vi "imp_test_v10_p1.vi"() -> ()   [LabVIEW 2014]
uses:
  <vilib>/LabVIEW Targets/FPGA/cRIO/shared/nicrio_ModuleControls/nicrio_cRIO-9237_DataRatesRing.ctl
  <vilib>/LabVIEW Targets/FPGA/cRIO/shared/nicrio_ModuleControls/nicrio_cRIO-9237_ExcitationVoltageRing.ctl
  <vilib>/rvi/FXPMathLib/FxpSinAndCos/subVIs/nifxpmath_SinAndCos_SimConfig.ctl
  <vilib>/rvi/Emulation/niFpgaGetClockAttributes.vi
  <vilib>/rvi/Emulation/niFpgaSctlEmulationGetInTimedLoop.vi
  <vilib>/rvi/Emulation/niFpgaEmulationReportErrorSimple.vi
  <vilib>/rvi/Emulation/niFpgaProcessEmulError.vi
  <vilib>/rvi/interface/RandomDataEmulation/nirviRandomDataMultiElementFPGAFIFO.vi
  <instcachedir>/0/nirviRandomDataMultiElementFPGAFIFO_AD0CFC12EF974623A9C2E4184BC062B2.lvgen/nirviRandomDataMultiElementFPGAFIFO_AD0CFC12EF974623A9C2E4184BC062B2_028.vi
  <vilib>/rvi/interface/RandomDataEmulation/niFpgaRandomDataHandleErrors.vi
  <vilib>/rvi/Emulation/niFpgaCriticalErrorInLSC.vi
  <vilib>/rvi/FXPMathLib/FxpSinAndCos/simVIs/DllFxpSinAndCosTemp_sub.vi
  <vilib>/rvi/eio/common/nirviEmuTemplateMethod_errors.vi
  <vilib>/rvi/eio/common/nirviEmuTemplatePropertySet_errors.vi
  <vilib>/rvi/DataTransferAndStorage/Container/XNode/niFpgaContainer.xnode
  <vilib>/rvi/interface/RandomDataEmulation/nirviRandomDataFpgaMultiElementTemplate.vi
  <vilib>/rvi/Analysis/measure/butterworth/XNode/niFpgaButterworthFilter.xnode
  <vilib>/rvi/FXPMathLib/FxpSinAndCos/XNode/nifxpmath_SinAndCos.xnode
  <vilib>/eio/EIONode/EIONode.xnode
  <vilib>/eio/EIOPropertyNode/EIOPropertyNode.xnode
  <vilib>/rvi/eio/common/nirviEmuTemplatePropertyGet_errors.vi
  <vilib>/rvi/eio/common/nirviEmuTemplatePropertyGet_noerrors.vi
  <vilib>/rvi/eio/common/nirviEmuTemplatePropertySet_noerrors.vi
panel:
  in  "F_Threshold_p":fxp<+,12,4>
  out "omega_p (Mavg)":fxp<+/-,36,13>
  out "Dp_d (Mavg)":fxp<+/-,36,13>
  out "omega_p2 (Mavg)":fxp<+/-,36,14>
  out "Dp2_d (Mavg)":fxp<+/-,36,14>
  in  "mt0_p2":u32
  out "Dp_d (Mavg w. f.)":fxp<+/-,36,14>
  in  "Dp_d (Mavg) coeff.":i32[](array[numeric])=[946630756, 63555534]
  out "omega_p (Mavg w. f)":fxp<+/-,36,14>
  in  "omega_P(Mavg) coeff.":i32[](array[numeric])=[946630756, 63555534]
  out "PID (kHz)":fxp<+/-,20,10>
  in  "Set 6":bool
  in  "Set 5":bool
  in  "Set 4":bool
  in  "Set 3":bool
  in  "Set 2":bool
  in  "Set 1":bool
  out "Dp1_d (T)":fxp<+/-,36,13>
  out "omega_p1 (T)":fxp<+/-,36,13>
  out "Dp2_d (T)":fxp<+/-,36,13>
  out "omega_p2 (T)":fxp<+/-,36,13>
  out "mt_omega_p2":u32
  out "Encoder Position_p2":i32
  out "D_p2":fxp<+/-,32,7>
  out "rad_p2":fxp<+/-,33,20>
  out "D_p1":fxp<+/-,32,7>
  out "rad_p1":fxp<+/-,33,20>
  out "Encoder Position_p1":i32
  out "Dp1_d (Mavg)":fxp<+/-,36,14>
  out "omega_p1 (Mavg)":fxp<+/-,36,14>
  in  "Dp_d_M_avg_Tc (uSec)":i32
  out "Dp_d (T)":fxp<+/-,36,13>
  out "omega_p (T)":fxp<+/-,36,13>
  in  "Vp. Est.":i16(ring) items=["T", "Mavg", "Mavg w. f."]
  in  "Mag. factor_p":fxp<+/-,20,3>
  in  "Mag. encoder_p":bool
  in  "Belt_out_p":fxp<+/-,7,7>
  in  "Belt_in_p":fxp<+/-,6,6>
  out "Fp_dc":fxp<+/-,32,10>
  in  "Zero_p":bool
  in  "mt0_p1":u32
  in  "Encoder reset":bool
  out "fpt_d":fxp<+/-,36,18>
  out "Dp_error_dd":fxp<+/-,36,16>
  out "Dp_error_d":fxp<+/-,33,8>
  in  "Dp_dd coeff.":i32[](array[numeric])=[946630756, 63555534]
  out "Dp_dd":fxp<+/-,36,25>
  out "dFp_PID":fxp<+/-,36,18>
  in  "dFp_PID coeff.":i32[](array[numeric])=[946630756, 63555534]
  out "fpt_i":fxp<+/-,34,18>
  in  "Bv_p":fxp<+/-,22,8>
  in  "Kv_p":fxp<+/-,22,8>
  out "Dp_error":fxp<+/-,22,7>
  out "Dpr_sin":fxp<+/-,22,7>
  in  "Sin offset_p":fxp<+/-,22,7>
  in  "Sin magnitude_p":fxp<+/-,21,6>
  out "Dpr_sin_dd":fxp<+/-,35,20>
  out "Dpr_sin_d":fxp<+/-,33,15>
  out "Sin omega_p":fxp<+/-,34,9>
  in  "Sin wave freq._p (Hz)":fxp<+/-,32,6>
  in  "Dpr_step":fxp<+/-,22,7>
  out "Dpr_for":fxp<+/-,22,7>
  in  "Command_p":i16(ring) items=["Step", "Sine"]
  in  "Ki_p":fxp<+/-,30,9>
  out "Fp_PID":fxp<+/-,36,16>
  in  "fp_tolorance":fxp<+,22,6>
  out "fp_tilde":fxp<+/-,33,10>
  in  "Kd_p":fxp<+/-,30,9>
  in  "Kp_p":fxp<+/-,32,13>
  out "Fr_p":fxp<+/-,32,10>
  in  "S/F coeff_p":fxp<+/-,25,-10>
  out "va_p":fxp<+/-,36,7>
  out "vb_p":fxp<+/-,37,8>
  out "vq_p_F":fxp<+/-,20,5> format="%.57g"
  out "vd_p_F":fxp<+/-,20,5>
  in  "dFp_add":bool
  in  "Stop motor_p":bool
  out "Force_p":fxp<+/-,32,10>
  in  "Strain selection_p":i16(ring) items=["Raw", "Avg.8", "Avg.8 w. filter"]
  out "Strain_p (Avg8 w. f)":fxp<+/-,36,8>
  in  "Strain_p Avg.8 coeff.":i32[](array[numeric])=[946630756, 63555534]
  out "Strain_p (Avg8)":fxp<+/-,36,4>
  out "Raw Strain_p":fxp<+/-,36,4>
  out "Mod6/AI3":fxp<+/-,36,4>
  in  "Strain gage reset_p":bool
  out "Dp_d (mm/s)":fxp<+/-,36,13>
  out "omega_p (rad/s)":fxp<+/-,36,13>
  out "mt_omega_p1":u32
  out "rad_p(NrTheta)":fxp<+/-,33,20>
  out "D_p(mm)":fxp<+/-,32,7>
  out "Encoder Position_p":i32
  in  "Encoder reset_p":bool
  out "Time now(s)":fxp<+,52,14>
  in  "Drive mode":i16(ring) items=["Backward", "Forward"]
  in  "Ini coe.":bool
  out "Loop rate (kHz)":fxp<+/-,36,7>
  in  "Stop (Strain)":bool
  in  "Excitation Voltage":T1 items=["2.5 Volts", "3.3 Volts", "5.0 Volts", "10.0 Volts", "External Excitation"]
  in  "Data Rate":T2=1 items=["50.000 kS/s (NI 9237)"=1, "25.000 kS/s (NI 9237)"=2, "16.667 kS/s (NI 9237)"=3, "12.500 kS/s (NI 9237)"=4, "10.000 kS/s (NI 9237)"=5, "8.333 kS/s (NI 9237)"=6, "7.143 kS/s (NI 9237)"=7, "6.250 kS/s (NI 9237)"=8, "5.556 kS/s (NI 9237)"=9, "5.000 kS/s (NI 9237)"=10, "4.545 kS/s (NI 9237)"=11, "4.167 kS/s (NI 9237)"=12, "3.846 kS/s (NI 9237)"=13, "3.571 kS/s (NI 9237)"=14, "3.333 kS/s (NI 9237)"=15, "3.125 kS/s (NI 9237)"=16, "2.941 kS/s (NI 9237)"=17, "2.778 kS/s (NI 9237)"=18, "2.632 kS/s (NI 9237)"=19, "2.500 kS/s (NI 9237)"=20, "2.381 kS/s (NI 9237)"=21, "2.273 kS/s (NI 9237)"=22, "2.174 kS/s (NI 9237)"=23, "2.083 kS/s (NI 9237)"=24, "2.000 kS/s (NI 9237)"=25, "1.923 kS/s (NI 9237)"=26, "1.852 kS/s (NI 9237)"=27, "1.786 kS/s (NI 9237)"=28, "1.724 kS/s (NI 9237)"=29, "1.667 kS/s (NI 9237)"=30, "1.613 kS/s (NI 9237)"=31]
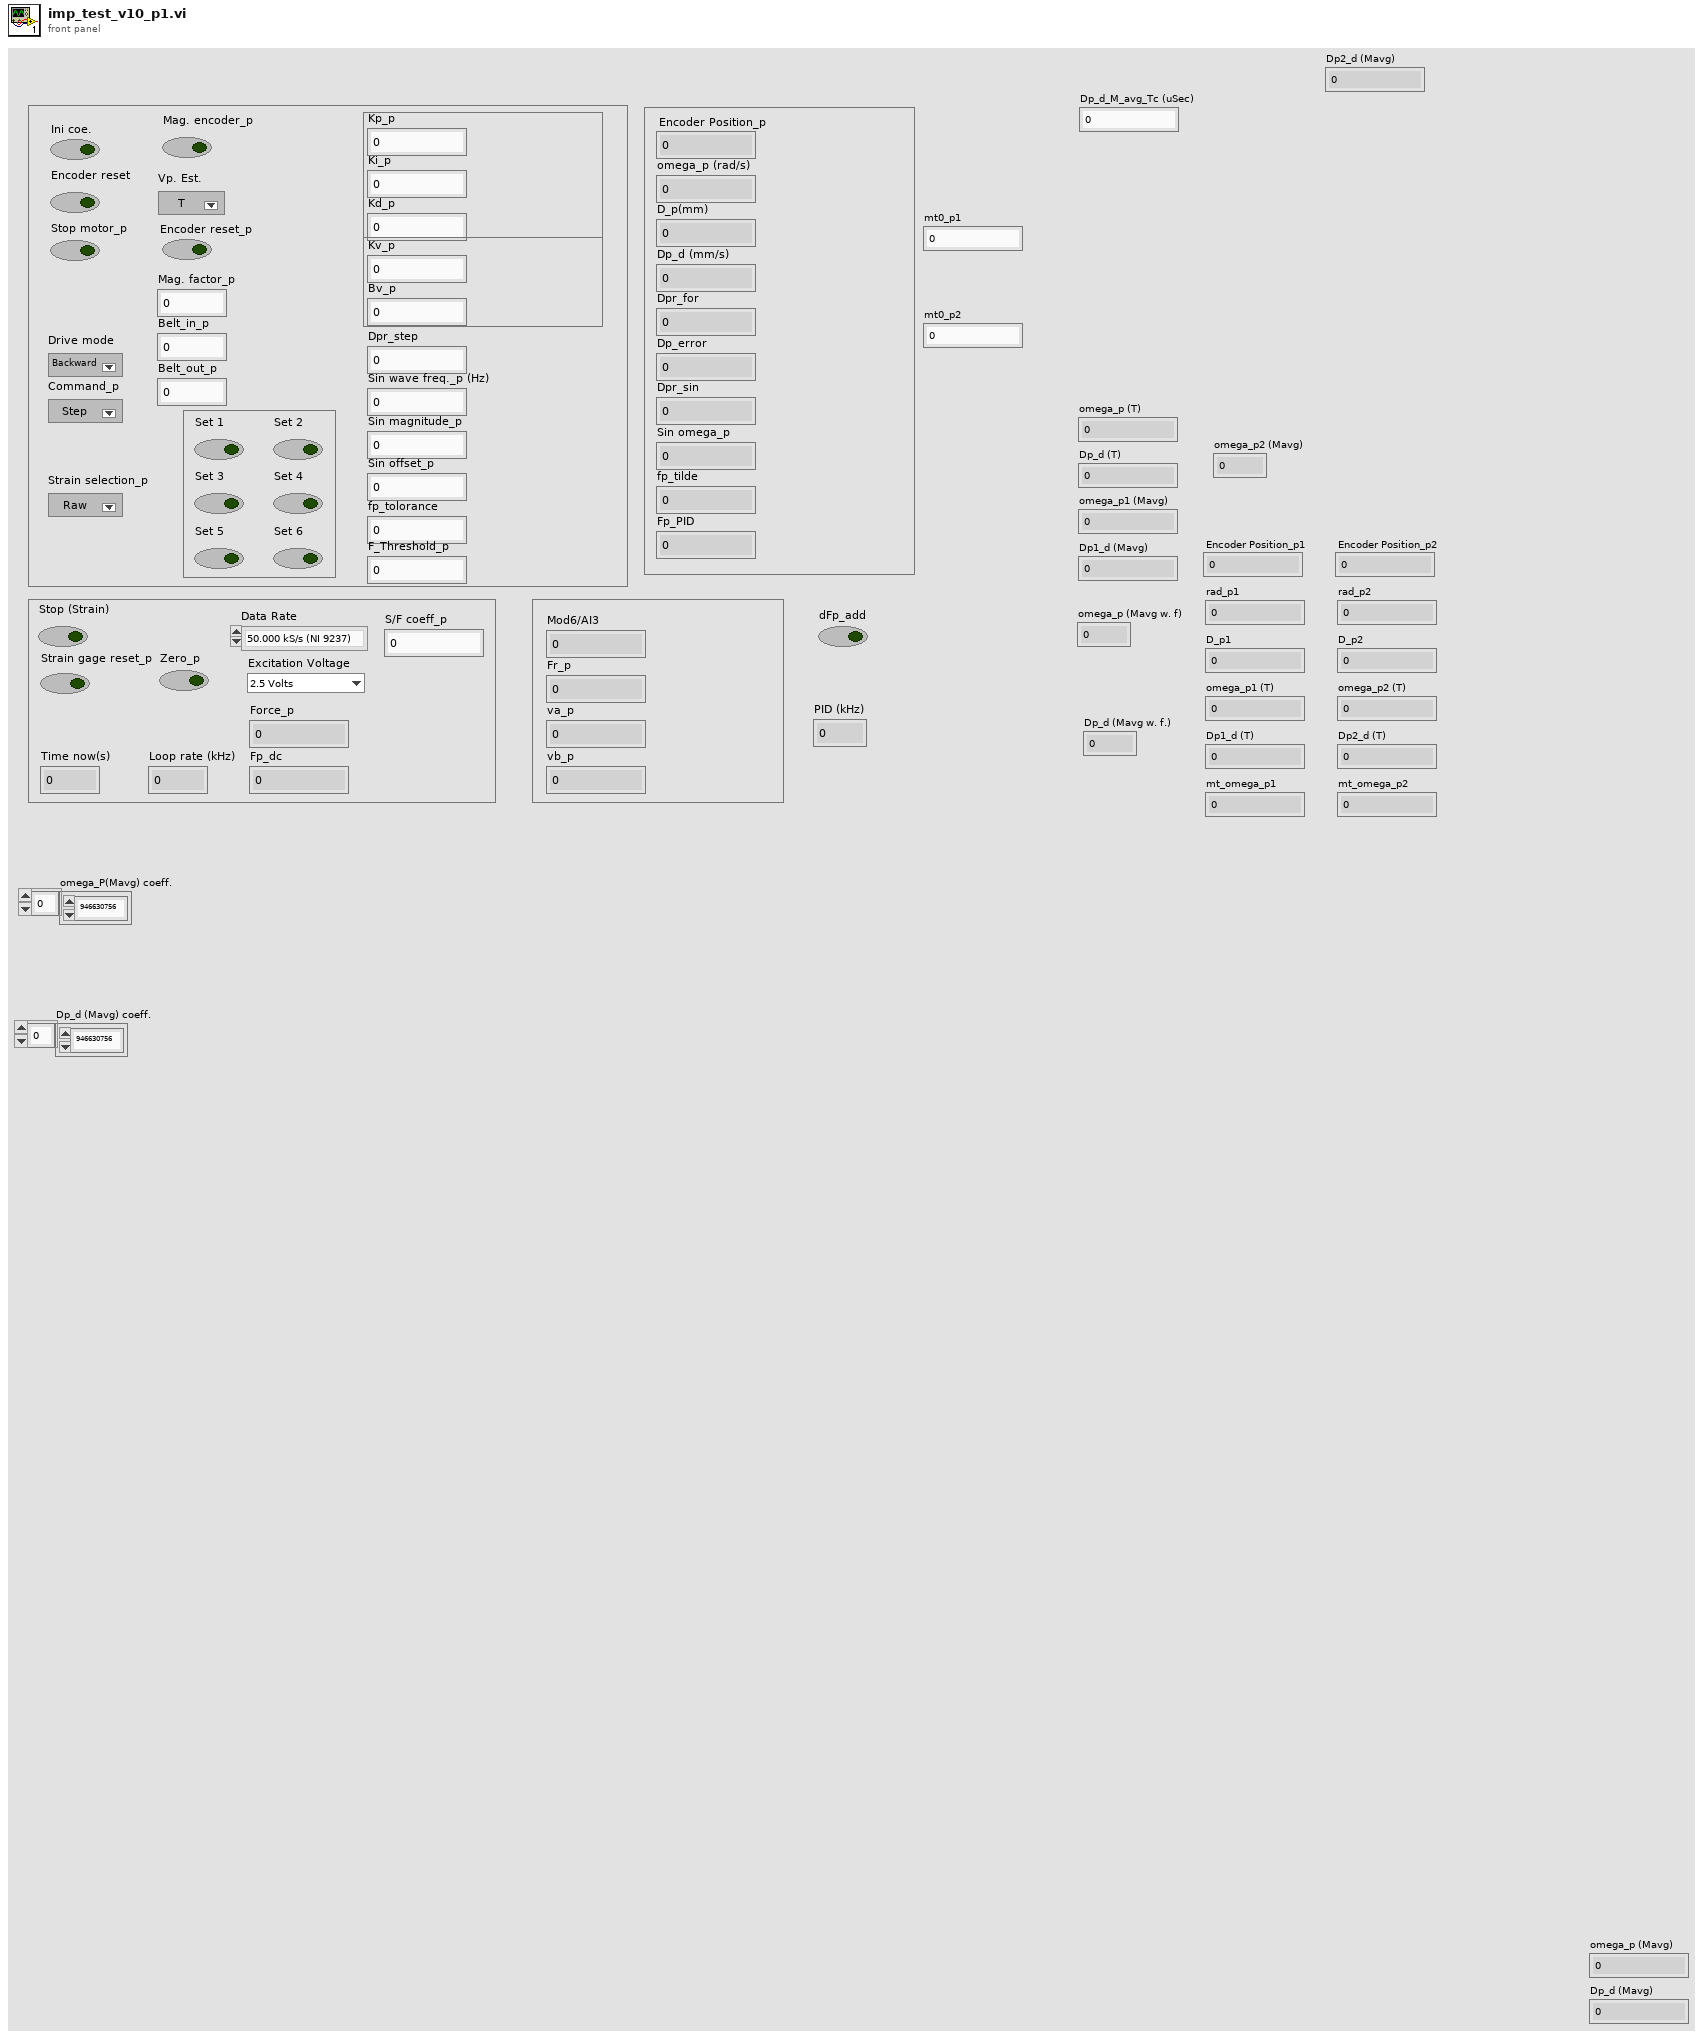
[diagram p1: front panel]
types:
  T1 = typedef "nicrio_cRIO-9237_ExcitationVoltageRing.ctl" = u8
  T2 = typedef "nicrio_cRIO-9237_DataRatesRing.ctl" = u8
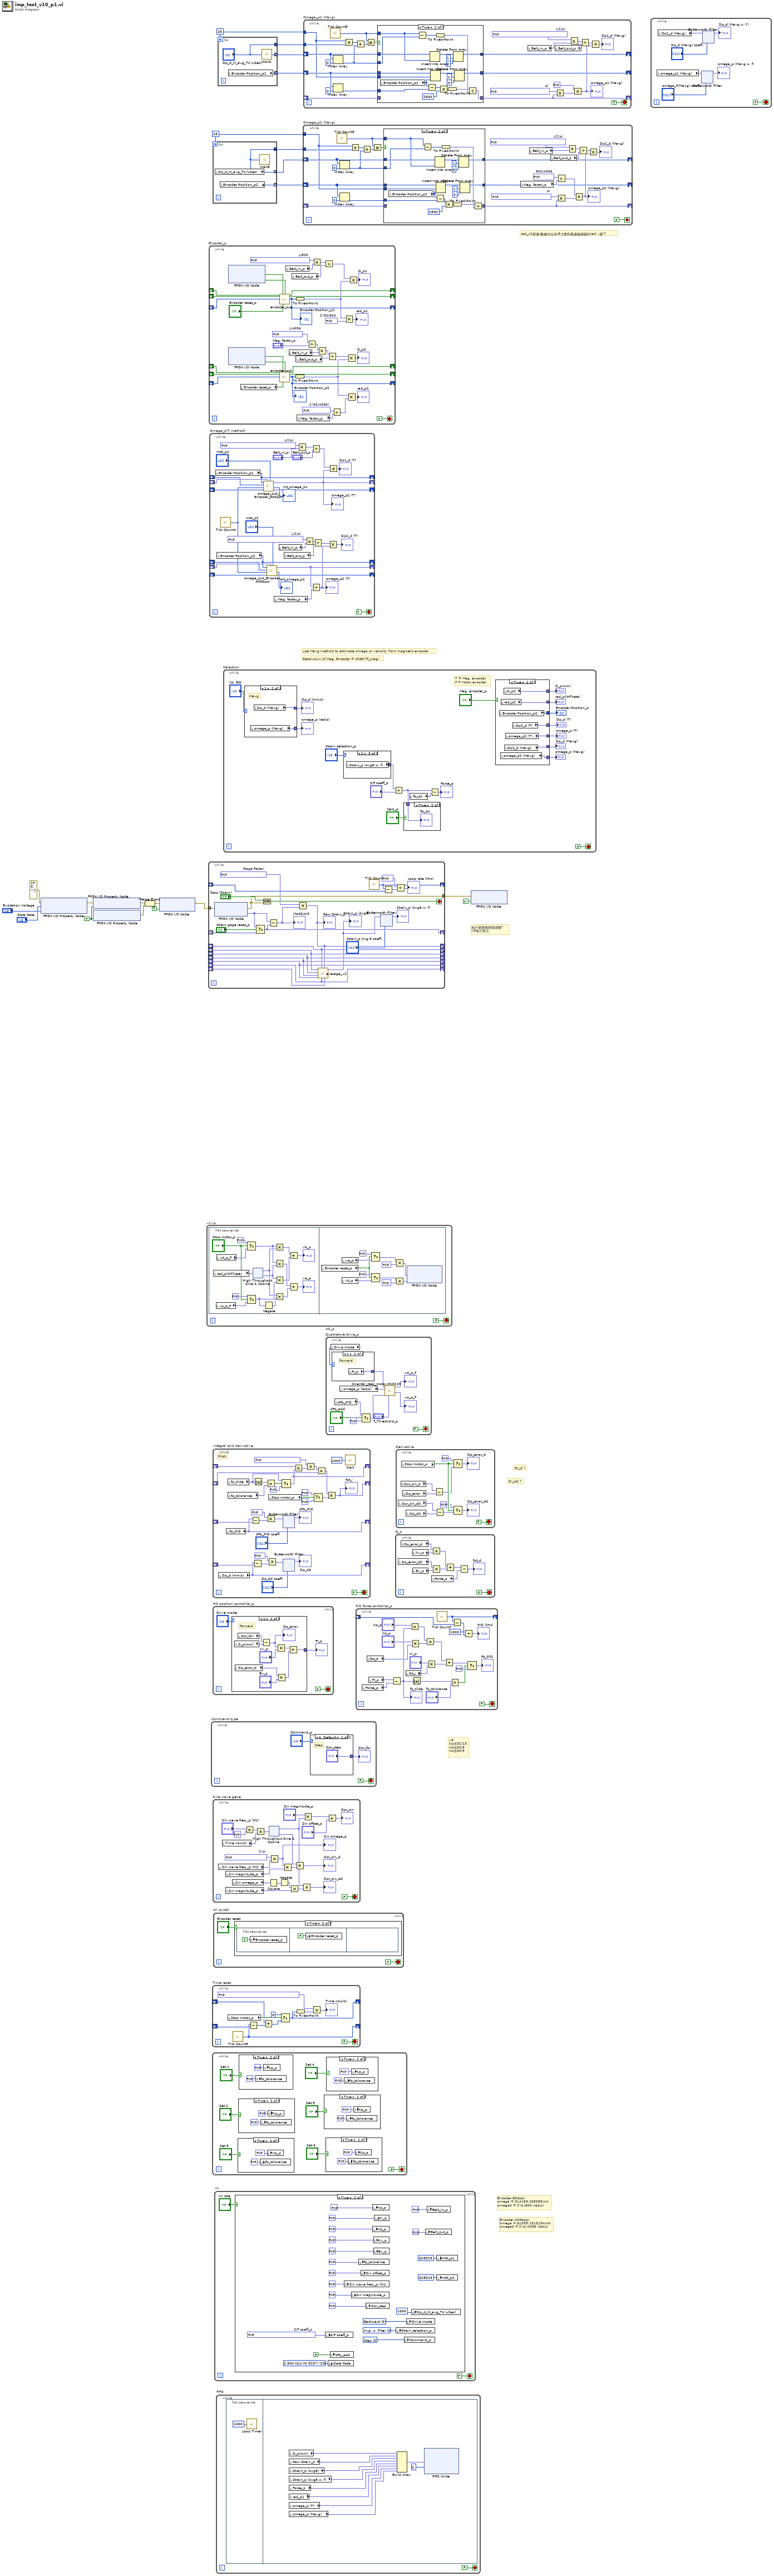
[diagram p0: block diagram]
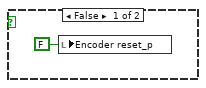
[diagram p10: hidden frame]
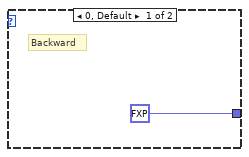
[diagram p11: hidden frame]
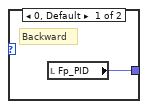
[diagram p12: hidden frame]
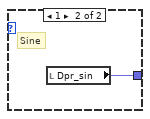
[diagram p13: hidden frame]
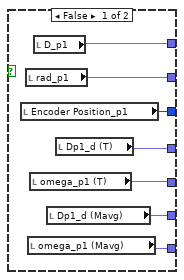
[diagram p14: hidden frame]
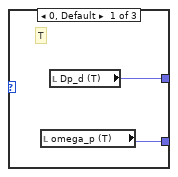
[diagram p15: hidden frame]
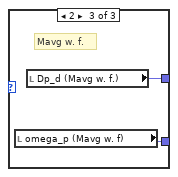
[diagram p16: hidden frame]
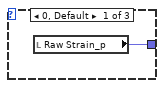
[diagram p18: hidden frame]
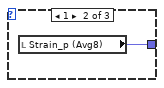
[diagram p19: hidden frame]
diagram:
  w2 = 25
  w8 = 25
  w13 = TRUE ("Half-Bridge Enable")
  # "rad_x2那邊:數據叫出來/8才會和馬達編碼器的rad一樣??"
  # "Encoder 4096ppr\nomega = 61359.2315154/mt\nomega0 = 2*pi/4096 (rad/s)"
  # "Encoder 800ppr\nomega = 314159.265359/mt\nomega0 = 2*pi/800 (rad/s)"
  # "v9\nKp改32/13\nKd改30/9\nKo改30/9"
  # "Resolutuin of Mag. Encoder = 4096*(F_mag)"
  # "use Mavg method to estimate omega or velocity from magnetic encoder"
  # "為什麼要寫兩個迴圈?\nv9後已修正"
  # "Dr_dd ?"
  # "Dr_d ?"
  n1 = xnode "FPGA I/O Property Node"("error in"=errorcluster {"status"=FALSE, "code"=0, "source"=""}, "Data Rate"="Data Rate", "Excitation Voltage"="Excitation Voltage") -> ("error out"=w18:errorcluster)  [unwired: 1 in, 1 out]
  n2 = xnode "FPGA I/O Property Node"("error in"=w18, "Half-Bridge Enable"=w13) -> ("error out"=w11:errorcluster)  [unwired: 1 in, 1 out]
  n3 = xnode "FPGA I/O Property Node"("Half-Bridge Enable"=w13) -> ("error out"=w10:errorcluster)  [unwired: 2 in, 1 out]
  n4 = Merge Errors(w11, w10) -> (w12:errorcluster)
  n5 = xnode "FPGA I/O Node"("error in"=w12, "Mod6/Start"=TRUE) -> ("error out"=w16:errorcluster)  [unwired: 1 in, 1 out]
  n6 = while "AO_p" {
    stop <- FALSE stop-if-true
    n7 = flat-sequence {
      frame #0 {
        n8 = local read "rad_p(NrTheta)"() -> (w33:fxp<+/-,33,20>)
        n9 = local read "vq_p_F"() -> (w34:fxp<+/-,20,5>)
        n10 = local read "vd_p_F"() -> (w36:fxp<+/-,20,5>)
        n11 = Select(t=fxp<+/-,20,5> 0.0, s="Stop motor_p", f=w36) -> (s? t:f=w25:fxp<+/-,20,5>)
        n12 = Select(t=fxp<+,1,1> 0.0, s="Stop motor_p", f=w34) -> (s? t:f=w24:fxp<+/-,20,5>)
        n13 = xnode "High Throughput Sine & Cosine"("x (pi)"=w33) -> ("sin(x)"=w27:fxp<+/-,16,2>, "cos(x)"=w26:fxp<+/-,16,2>)
        n14 = Negate(x=w24) -> (-x=w32:fxp<+/-,21,6>)
        n15 = Multiply(x=w25, y=w27) -> (x*y=w31:fxp<+/-,36,7>)
        n16 = Multiply(x=w25, y=w26) -> (x*y=w29:fxp<+/-,36,7>)
        n17 = Multiply(x=w26, y=w24) -> (x*y=w30:fxp<+/-,36,7>)
        n18 = Multiply(x=w27, y=w32) -> (x*y=w28:fxp<+/-,35,6>)
        n19 = Add(x=w31, y=w30) -> (x+y=→"vb_p":fxp<+/-,37,8>)
        n20 = Add(x=w29, y=w28) -> (x+y=→"va_p":fxp<+/-,36,7>)
      }
      frame #1 {
        n21 = local read "Encoder reset_p"() -> (w69:bool)
        n22 = local read "vb_p"() -> (w70:fxp<+/-,37,8>)
        n23 = local read "va_p"() -> (w71:fxp<+/-,36,7>)
        n24 = Select(t=fxp<+,2,2> 3.0, s=w69, f=w71) -> (s? t:f=w77:fxp<+/-,36,7>)
        n25 = Select(t=fxp<+,1,1> 0.0, s=w69, f=w70) -> (s? t:f=w76:fxp<+/-,37,8>)
        n26 = Multiply(x=w77, y=fxp<+/-,1,0> -0.5) -> (x*y=w72:fxp<+/-,36,6>)
        n27 = Multiply(x=w76, y=fxp<+/-,1,0> -0.5) -> (x*y=w73:fxp<+/-,36,6>)
        n28 = xnode "FPGA I/O Node"("Mod8/AO0"=w72, "Mod8/AO1"=w73) -> ()  [unwired: 2 in, 2 out]
      }
    }
  }
  n29 = while {
    tunnel: [w80] -> w9
    shift-right: [w104] -> _
    shift-left: _ -> [w105]
    tunnel: w16 -> [w100]
    shift-right: [w96] -> _
    shift-left: _ -> [w97]
    shift-right: [w92] -> _
    shift-left: _ -> [w91]
    shift-right: [w91] -> _
    shift-left: _ -> [w90]
    shift-right: [w90] -> _
    shift-left: _ -> [w89]
    shift-right: [w89] -> _
    shift-left: _ -> [w88]
    shift-right: [w88] -> _
    shift-left: _ -> [w87]
    shift-right: [w87] -> _
    shift-left: _ -> [w86]
    shift-right: [w86] -> _
    shift-left: _ -> [w85]
    stop <- w99 stop-if-true
    w94 = fxp<+,20,2> 2.115001678466797  # Gage Factor
    n30 = xnode "FPGA I/O Node"("error in"=w100) -> ("error out"=w80:errorcluster, "Mod6/AI3"=w95:fxp<+/-,24,-4>)  [unwired: 1 in, 1 out]
    n31 = Select(t=w95, s="Strain gage reset_p", f=w97) -> (s? t:f=w96:fxp<+/-,24,-4>)
    n32 = Or(x="Stop (Strain)", y=w80) -> (x .or. y?=w99:bool)
    n33 = Subtract(x=w95, y=w96) -> (x-y=w93:fxp<+/-,30,-3>)
    "Mod6/AI3" <- w93
    n34 = Multiply(x=w94, y=w93) -> (x*y=w92:fxp<+/-,50,-1>)
    "Raw Strain_p" <- w92
    n35 = call "average_v2.vi"("Numeric 8"=w85, "Numeric"=w92, "Numeric 7"=w86, "Numeric 2"=w91, "Numeric 6"=w87, "Numeric 5"=w88, "Numeric 4"=w89, "Numeric 3"=w90) -> ("Mean (8pt)"=w84:fxp<+/-,32,4>)  [unwired: 1 in, 2 out]
    "Strain_p (Avg8)" <- w84
    n36 = call "Tick Count"() -> ("Tick Count(uSec)"=w104:u32)
    n37 = xnode "Butterworth Filter"("input data"=w84, "scaled coefficients"="Strain_p Avg.8 coeff.") -> ("output data"=→"Strain_p (Avg8 w. f)":fxp<+/-,36,8>)  [unwired: 1 in]
    n38 = Subtract(x=w104, y=w105) -> (x-y=w103:fxp<+/-,32,16>)
    n39 = Divide(x=fxp<+,7,10> 1000.0, y=w103) -> (x/y=→"Loop rate (kHz)":fxp<+/-,40,27>)
  }
  n40 = while "Encoder_p" {
    shift-right: [w151] -> _
    shift-left: _ -> [w150]
    shift-right: [w152] -> _
    shift-left: _ -> [w149]
    shift-right: [w146] -> _
    shift-left: _ -> [w148]
    shift-right: [w137] -> _
    shift-left: _ -> [w136]
    shift-right: [w138] -> _
    shift-left: _ -> [w139]
    shift-right: [w133] -> _
    shift-left: _ -> [w134]
    stop <- FALSE stop-if-true
    w129 = fxp<+/-,20,-5> 0.00048828125  # L/4096
    w127 = fxp<+/-,16,1> 0.0244140625  # 2*50/4096)
    w145 = fxp<+/-,20,-5> 0.002499997615814209  # L/800
    w119 = fxp<+/-,16,1> 0.125  # 2*50/800
    n41 = xnode "FPGA I/O Node"() -> ("Mod7/DIO0"=w154:bool, "Mod7/DIO1"=w153:bool)  [unwired: 2 in, 2 out]
    n42 = xnode "FPGA I/O Node"() -> ("Mod7/DIO4"=w141:bool, "Mod7/DIO5"=w140:bool)  [unwired: 2 in, 2 out]
    n43 = local read "Encoder reset_p"() -> (w135:bool)
    n44 = call "encoder_sub.vi"("A_pre"=w150, "B_pre"=w149, "Encoder Position_pre"=w148, "A input"=w154, "Encoder Position Reset"="Encoder reset_p", "B input"=w153) -> ("A"=w151:bool, "B"=w152:bool, "Encoder Position (Counts)"=w146:i32)  [unwired: 19 in]
    "Encoder Position_p1" <- w146
    n45 = call "encoder_sub.vi"("A_pre"=w136, "B_pre"=w139, "Encoder Position_pre"=w134, "A input"=w141, "Encoder Position Reset"=w135, "B input"=w140) -> ("A"=w137:bool, "B"=w138:bool, "Encoder Position (Counts)"=w133:i32)  [unwired: 19 in]
    "Encoder Position_p2" <- w133
    n46 = local read "Belt_in_p"() -> (w144:fxp<+/-,6,6>)
    n47 = local read "Belt_in_p"() -> (w130:fxp<+/-,6,6>)
    n48 = local read "Belt_out_p"() -> (w142:fxp<+/-,7,7>)
    n49 = To Fixed-Point(number=w133) -> (fixed-point=w115:fxp<+/-,32,32>)  [unwired: 1 in]
    n50 = To Fixed-Point(number=w146) -> (fixed-point=w120:fxp<+/-,32,32>)  [unwired: 1 in]
    n51 = local read "Belt_out_p"() -> (w132:fxp<+/-,7,7>)
    n52 = local read "Mag. factor_p"() -> (w126:fxp<+/-,20,3>)
    n53 = Divide(x=w129, y="Mag. factor_p") -> (x/y=w128:fxp<+/-,41,13>)
    n54 = Multiply(x=w145, y=w144) -> (x*y=w143:fxp<+/-,26,1>)
    n55 = Multiply(x=w128, y=w130) -> (x*y=w131:fxp<+/-,46,18>)
    n56 = Divide(x=w143, y=w142) -> (x/y=w122:fxp<+/-,33,1>)
    n57 = Divide(x=w131, y=w132) -> (x/y=w117:fxp<+/-,53,18>)
    n58 = Divide(x=w127, y=w126) -> (x/y=w114:fxp<+/-,37,5>)
    n59 = Multiply(x=w120, y=w119) -> (x*y=→"rad_p1":fxp<+/-,33,20>)
    n60 = Multiply(x=w117, y=w115) -> (x*y=→"D_p2":fxp<+/-,37,7>)
    n61 = Multiply(x=w115, y=w114) -> (x*y=→"rad_p2":fxp<+/-,46,16>)
    n62 = Multiply(x=w122, y=w120) -> (x*y=→"D_p1":fxp<+/-,32,7>)
  }
  n63 = while "Omega_p(T method)" {
    shift-right: [w186] -> _
    shift-left: _ -> [w184]
    shift-right: [w167] -> _
    shift-left: _ -> [w185]
    shift-right: [w182] -> _
    shift-left: _ -> [w183]
    shift-right: [w160] -> _
    shift-left: _ -> [w159]
    shift-right: [w155] -> _
    shift-left: _ -> [w157]
    shift-right: [w163] -> _
    shift-left: _ -> [w162]
    stop <- FALSE stop-if-true
    w174 = fxp<+/-,32,0> 0.3183098859153688  # L/2/pi
    w179 = fxp<+/-,32,0> 0.3183098859153688  # L/2/pi
    n64 = local read "Encoder Position_p1"() -> (w186:i32)
    n65 = local read "Encoder Position_p2"() -> (w160:i32)
    n66 = call "Tick Count4"() -> ("Tick Count(Ticks)"=w161:u32)
    n67 = call "omega_sub_Encoder_800ppr.vi"("mt0"="mt0_p1", "omega_pre"=w185, "ticks_m_pre"=w183, "ticks"=w161, "count_pre"=w184, "count"=w186) -> ("ticks_m"=w182:u32, "mt"=→"mt_omega_p1":u32, "omega"=w167:fxp<+/-,36,13>)  [unwired: 3 in]
    "omega_p1 (T)" <- w167
    n68 = call "omega_sub_Encoder_4096ppr.vi"("mt0"="mt0_p2", "omega_pre"=w157, "ticks_m_pre"=w162, "ticks"=w161, "count_pre"=w159, "count"=w160) -> ("ticks_m"=w163:u32, "mt"=→"mt_omega_p2":u32, "omega"=w155:fxp<+/-,36,13>)  [unwired: 3 in]
    n69 = local read "Mag. factor_p"() -> (w175:fxp<+/-,20,3>)
    n70 = local read "Belt_in_p"() -> (w172:fxp<+/-,6,6>)
    n71 = local read "Belt_out_p"() -> (w171:fxp<+/-,7,7>)
    n72 = Multiply(x=w179, y="Belt_in_p") -> (x*y=w177:fxp<+/-,38,6>)
    n73 = Multiply(x=w174, y=w172) -> (x*y=w173:fxp<+/-,38,6>)
    n74 = Divide(x=w177, y="Belt_out_p") -> (x/y=w168:fxp<+/-,20,1>)
    n75 = Divide(x=w155, y=w175) -> (x/y=w156:fxp<+/-,57,31>)
    "omega_p2 (T)" <- w156
    n76 = Divide(x=w173, y=w171) -> (x/y=w166:fxp<+/-,45,6>)
    n77 = Multiply(x=w166, y=w156) -> (x*y=→"Dp2_d (T)":fxp<+/-,36,13>)
    n78 = Multiply(x=w168, y=w167) -> (x*y=→"Dp1_d (T)":fxp<+/-,36,13>)
  }
  n79 = while "Command type" {
    stop <- FALSE stop-if-true
    n80 = case shown="0, Default" "Command_p" {
      tunnel: ["Dpr_step" w191] -> w188
      frame 0, Default {
        # "Step"
      }
      frame 1 {
        # "Sine"
        n81 = local read "Dpr_sin"() -> (w191:fxp<+/-,22,7>)
      }
    }
    "Dpr_for" <- w188
  }
  n82 = while "Time reset" {
    shift-right: [w201] -> _
    shift-left: _ -> [w202]
    shift-right: [w196] -> _
    shift-left: _ -> [w197]
    stop <- FALSE stop-if-true
    n83 = local read "Stop motor_p"() -> (w203:bool)
    n84 = call "Tick Count3"() -> ("Tick Count(uSec)"=w201:u32)
    n85 = Subtract(x=w201, y=w202) -> (x-y=w200:u32)
    n86 = Add(x=w197, y=w200) -> (x+y=w199:u32)
    n87 = Select(t=u32 0, s=w203, f=w199) -> (s? t:f=w196:u32)
    n88 = To Fixed-Point(number=w196) -> (fixed-point=w195:fxp<+,32,32>)  [unwired: 1 in]
    n89 = Multiply(x=fxp<+,20,-18> 1.0000003385357559e-06, y=w195) -> (x*y=→"Time now(s)":fxp<+,52,14>)
  }
  n90 = while {
    stop <- FALSE stop-if-true
    n91 = case shown="True" "Set 3" {
      frame False {
      }
      frame True {
        n92 = local write "fp_tolorance"(fxp<+,22,6> 3.0 ("fp_tolorance")) -> ()
        n93 = local write "Kp_p"(fxp<+/-,36,9> 100.0 ("Kp_p")) -> ()
      }
    }
    n94 = case shown="True" "Set 2" {
      frame False {
      }
      frame True {
        n95 = local write "fp_tolorance"(fxp<+,22,6> 1.5 ("fp_tolorance")) -> ()
        n96 = local write "Kp_p"(fxp<+/-,36,9> 50.0 ("Kp_p")) -> ()
      }
    }
    n97 = case shown="True" "Set 1" {
      frame False {
      }
      frame True {
        n98 = local write "fp_tolorance"(fxp<+,22,6> 3.0 ("fp_tolorance")) -> ()
        n99 = local write "Kp_p"(fxp<+/-,36,9> 50.0 ("Kp_p")) -> ()
      }
    }
    n100 = case shown="True" "Set 5" {
      frame False {
      }
      frame True {
        n101 = local write "fp_tolorance"(fxp<+,22,6> 3.0 ("fp_tolorance")) -> ()
        n102 = local write "Kp_p"(fxp<+/-,36,9> 150.0 ("Kp_p")) -> ()
      }
    }
    n103 = case shown="True" "Set 6" {
      frame False {
      }
      frame True {
        n104 = local write "fp_tolorance"(fxp<+,22,6> 1.5 ("fp_tolorance")) -> ()
        n105 = local write "Kp_p"(fxp<+/-,36,9> 150.0 ("Kp_p")) -> ()
      }
    }
    n106 = case shown="True" "Set 4" {
      frame False {
      }
      frame True {
        n107 = local write "fp_tolorance"(fxp<+,22,6> 1.5 ("fp_tolorance")) -> ()
        n108 = local write "Kp_p"(fxp<+/-,36,9> 100.0 ("Kp_p")) -> ()
      }
    }
  }
  n109 = for {
    N: w2 -> [_]
    tunnel: [w224] -> w4 mode=indexing
    tunnel: [w223] -> w3 mode=indexing
    tunnel: [w223] -> w1
    n110 = local read "Dp_d_M_avg_Tc (uSec)"() -> (w223:i32)
    n111 = local read "Encoder Position_p2"() -> (w224:i32)
    n112 = call "Wait5"("Count(uSec)"=w223) -> ()  [unwired: 1 out]
  }
  n113 = while "Sine wave gene" {
    stop <- FALSE stop-if-true
    w230 = fxp<+,20,3> 6.2831878662109375  # 2*pi
    n114 = local read "Sin wave freq._p (Hz)"() -> (w226:fxp<+/-,32,6>)
    n115 = local read "Time now(s)"() -> (w244:fxp<+,52,14>)
    n116 = local read "Sin magnitude_p"() -> (w227:fxp<+/-,21,6>)
    n117 = local read "Sin magnitude_p"() -> (w229:fxp<+/-,21,6>)
    n118 = local read "Sin omega_p"() -> (w228:fxp<+/-,34,9>)
    n119 = Multiply(x="Sin wave freq._p (Hz)", y=fxp<+/-,10,3> 2.0) -> (x*y=w248:fxp<+/-,42,9>)
    n120 = Multiply(x=w248, y=w244) -> (x*y=w245:fxp<+/-,41,19>)
    n121 = Square(x=w228) -> (x^2=w240:fxp<+,34,18>)
    n122 = xnode "High Throughput Sine & Cosine"("x (pi)"=w245) -> ("sin(x)"=w231:fxp<+/-,16,2>, "cos(x)"=w236:fxp<+/-,16,2>)
    n123 = Multiply(x=w230, y=w226) -> (x*y=w243:fxp<+/-,34,9>)
    "Sin omega_p" <- w243
    n124 = Negate(x=w240) -> (-x=w239:fxp<+/-,35,19>)
    n125 = Multiply(x=w243, y=w227) -> (x*y=w242:fxp<+/-,33,15>)
    n126 = Multiply(x=w239, y=w229) -> (x*y=w238:fxp<+/-,35,19>)
    n127 = Multiply(x=w236, y=w242) -> (x*y=→"Dpr_sin_d":fxp<+/-,33,15>)
    n128 = Multiply(x=w231, y=w238) -> (x*y=→"Dpr_sin_dd":fxp<+/-,35,20>)
    n129 = Multiply(x="Sin magnitude_p", y=w231) -> (x*y=w234:fxp<+/-,37,8>)
    n130 = Add(x=w234, y="Sin offset_p") -> (x+y=→"Dpr_sin":fxp<+/-,37,8>)
  }
  n131 = while "Integral and derivative" {
    shift-right: [w302] -> _
    shift-left: _ -> [w305]
    shift-right: [w295] -> _
    shift-left: _ -> [w294]
    shift-right: [w289] -> _
    shift-left: _ -> [w288]
    shift-right: [w284] -> _
    shift-left: _ -> [w285]
    stop <- FALSE stop-if-true
    # "Pitch"
    n132 = local read "Dp_d (mm/s)"() -> (w284:fxp<+/-,36,13>)
    n133 = local read "Fp_PID"() -> (w289:fxp<+/-,36,16>)
    n134 = local read "fp_tilde"() -> (w306:fxp<+/-,33,10>)
    n135 = local read "fp_tolorance"() -> (w309:fxp<+,22,6>)
    n136 = Subtract(x=w289, y=w288) -> (x-y=w293:fxp<+/-,37,17>)
    n137 = Subtract(x=w284, y=w285) -> (x-y=w286:fxp<+/-,37,14>)
    n138 = Absolute Value(x=w306) -> (abs(x)=w310:fxp<+,33,10>)
    n139 = Greater?(x=w310, y=w309) -> (0:w308:bool)
    n140 = Multiply(x=fxp<+,7,10> 1000.0, y=w293) -> (x*y=w291:fxp<+/-,32,18>)
    n141 = Multiply(x=fxp<+,7,10> 1000.0, y=w286) -> (x*y=w282:fxp<+/-,36,21>)
    n142 = local read "Stop motor_p"() -> (w297:bool)
    n143 = Select(t=w306, s=w308, f=fxp<+,1,1> 0.0) -> (s? t:f=w302:fxp<+/-,33,10>)
    n144 = xnode "Butterworth Filter"("input data"=w291, "scaled coefficients"="dFp_PID coeff.") -> ("output data"=→"dFp_PID":fxp<+/-,36,22>)  [unwired: 1 in]
    n145 = xnode "Butterworth Filter"("input data"=w282, "scaled coefficients"="Dp_dd coeff.") -> ("output data"=→"Dp_dd":fxp<+/-,36,25>)  [unwired: 1 in]
    n146 = Multiply(x=w305, y=w302) -> (x*y=w304:fxp<+/-,34,12>)
    n147 = Multiply(x=fxp<+/-,30,12> 0.000499725341796875, y=w304) -> (x*y=w301:fxp<+/-,34,10>)
    n148 = Select(t=fxp<+,1,1> 0.0, s=w297, f=fxp<+,1,1> 1.0) -> (s? t:f=w299:fxp<+,1,1>)
    n149 = Add(x=w301, y=w294) -> (x+y=w300:fxp<+/-,36,16>)
    n150 = Multiply(x=w300, y=w299) -> (x*y=w295:fxp<+/-,34,18>)
    "fpt_i" <- w295
    n151 = call "Wait"("Count(uSec)"=u32 1000) -> ()  [unwired: 1 out]
  }
  n152 = while "PD position controller_p" {
    stop <- FALSE stop-if-true
    n153 = case shown="1" "Drive mode" {
      tunnel: [fxp<+/-,62,19> 0.0 w333] -> w330
      frame 0, Default {
        # "Backward"
      }
      frame 1 {
        # "Forward"
        n154 = local read "D_p(mm)"() -> (w340:fxp<+/-,32,7>)
        n155 = local read "Dp_error_d"() -> (w332:fxp<+/-,33,8>)
        n156 = local read "Dpr_for"() -> (w339:fxp<+/-,22,7>)
        n157 = Subtract(x=w339, y=w340) -> (x-y=w338:fxp<+/-,33,8>)
        "Dp_error" <- w338
        n158 = Multiply(x=w338, y="Kv_p") -> (x*y=w335:fxp<+/-,54,15>)
        n159 = Multiply(x=w332, y="Bv_p") -> (x*y=w334:fxp<+/-,55,16>)
        n160 = Add(x=w335, y=w334) -> (x+y=w333:fxp<+/-,55,16>)
      }
    }
    "Fr_p" <- w330
  }
  n161 = while "All switch" {
    stop <- FALSE stop-if-true
    n162 = case shown="True" "Encoder reset" {
      frame False {
        n163 = local write "Encoder reset_p"(FALSE ("Encoder reset_p")) -> ()
      }
      frame True {
        n164 = flat-sequence {
          frame #0 {
            n165 = local write "Encoder reset_p"(TRUE ("Encoder reset_p")) -> ()
          }
          frame #1 {
            n166 = local write "Encoder reset_p"(FALSE ("Encoder reset_p")) -> ()
          }
          frame #2 {
          }
        }
      }
    }
  }
  n167 = while "Ini" {
    stop <- FALSE stop-if-true
    n168 = case shown="True" "Ini coe." {
      frame False {
      }
      frame True {
        w350 = T2 20 items=["50.000 kS/s (NI 9237)"=1, "25.000 kS/s (NI 9237)"=2, "16.667 kS/s (NI 9237)"=3, "12.500 kS/s (NI 9237)"=4, "10.000 kS/s (NI 9237)"=5, "8.333 kS/s (NI 9237)"=6, "7.143 kS/s (NI 9237)"=7, "6.250 kS/s (NI 9237)"=8, "5.556 kS/s (NI 9237)"=9, "5.000 kS/s (NI 9237)"=10, "4.545 kS/s (NI 9237)"=11, "4.167 kS/s (NI 9237)"=12, "3.846 kS/s (NI 9237)"=13, "3.571 kS/s (NI 9237)"=14, "3.333 kS/s (NI 9237)"=15, "3.125 kS/s (NI 9237)"=16, "2.941 kS/s (NI 9237)"=17, "2.778 kS/s (NI 9237)"=18, "2.632 kS/s (NI 9237)"=19, "2.500 kS/s (NI 9237)"=20, "2.381 kS/s (NI 9237)"=21, "2.273 kS/s (NI 9237)"=22, "2.174 kS/s (NI 9237)"=23, "2.083 kS/s (NI 9237)"=24, "2.000 kS/s (NI 9237)"=25, "1.923 kS/s (NI 9237)"=26, "1.852 kS/s (NI 9237)"=27, "1.786 kS/s (NI 9237)"=28, "1.724 kS/s (NI 9237)"=29, "1.667 kS/s (NI 9237)"=30, "1.613 kS/s (NI 9237)"=31] ("Data Rate")
        w365 = i16 0 items=["Step", "Sine"] ("Command_p")
        w366 = i16 2 items=["Raw", "Avg.", "Avg. w. filter"] ("Strain selection_p")
        w367 = fxp<+/-,25,-10> 5.851034075021744e-07  # S/F coeff_p
        w368 = i16 0 items=["Backward", "Forward"] ("Drive mode")
        n169 = local write "S/F coeff_p"(w367) -> ()
        n170 = local write "Data Rate"(w350) -> ()
        n171 = local write "dFp_add"(FALSE ("dFp_add")) -> ()
        n172 = local write "Sin wave freq._p (Hz)"(fxp<+/-,32,6> 1.0 ("Sin wave freq._p (Hz)")) -> ()
        n173 = local write "Sin magnitude_p"(fxp<+/-,21,6> 5.0 ("Sin magnitude_p")) -> ()
        n174 = local write "fp_tolorance"(fxp<+,22,6> 5.0 ("fp_tolorance")) -> ()
        n175 = local write "Sin offset_p"(fxp<+/-,22,7> 0.0 ("Sin offset_p")) -> ()
        n176 = local write "Dpr_step"(fxp<+/-,22,7> 0.0 ("Dpr_step")) -> ()
        n177 = local write "Kp_p"(fxp<+/-,36,9> 30.0 ("Kp_p")) -> ()
        n178 = local write "Kd_p"(fxp<+/-,36,9> 0.0 ("Kd_p")) -> ()
        n179 = local write "Kv_p"(fxp<+/-,22,8> 0.0 ("Kv_p")) -> ()
        n180 = local write "Bv_p"(fxp<+/-,22,8> 0.0 ("Bv_p")) -> ()
        n181 = local write "Ki_p"(fxp<+/-,36,9> 0.0 ("Ki_p")) -> ()
        n182 = local write "Strain selection_p"(w366) -> ()
        n183 = local write "Command_p"(w365) -> ()
        n184 = local write "Drive mode"(w368) -> ()
        n185 = local write "Dp_d_M_avg_Tc (uSec)"(u32 1000 ("D_d_M_avg_Tc (uSec)")) -> ()
        n186 = local write "Belt_out_p"(fxp<+/-,7,7> 36.0 ("Belt_op")) -> ()
        n187 = local write "Belt_in_p"(fxp<+/-,6,6> 16.0 ("Belt_mp")) -> ()
        n188 = local write "mt0_p1"(u32 628319 ("mt0_p1")) -> ()
        n189 = local write "mt0_p2"(u32 628319 ("mt0_p2")) -> ()
      }
    }
  }
  n190 = while "FIFO" {
    stop <- FALSE stop-if-true
    n191 = flat-sequence {
      frame #0 {
        n192 = call "Loop Timer"("Count(uSec)"=u32 1000) -> ()  [unwired: 1 out]
      }
      frame #1 {
        n193 = local read "D_p(mm)"() -> (w378:fxp<+/-,32,7>)
        n194 = local read "Raw Strain_p"() -> (w377:fxp<+/-,36,4>)
        n195 = local read "Strain_p (Avg8)"() -> (w376:fxp<+/-,36,4>)
        n196 = local read "Strain_p (Avg8 w. f)"() -> (w375:fxp<+/-,36,8>)
        n197 = local read "Force_p"() -> (w374:fxp<+/-,32,10>)
        n198 = local read "rad_p1"() -> (w373:fxp<+/-,33,20>)
        n199 = local read "omega_p (T)"() -> (w372:fxp<+/-,36,13>)
        n200 = local read "omega_p (Mavg)"() -> (w371:fxp<+/-,36,13>)
        n201 = Build Array(w378, w377, w376, w375, w374, w373, w372, w371) -> (w379:fxp<+/-,52,20>[])
        n202 = xnode ("FIFO Write")("Element"=w379, "Timeout"=0) -> ()  [unwired: 1 in, 2 out]
      }
    }
  }
  n203 = for {
    N: w8 -> [_]
    tunnel: ["Dp_d_M_avg_Tc (uSec)"] -> w5
    tunnel: [w382] -> w7 mode=indexing
    tunnel: [w381] -> w6 mode=indexing
    n204 = local read "Encoder Position_p1"() -> (w381:i32)
    n205 = call "Wait2"("Count(uSec)"="Dp_d_M_avg_Tc (uSec)") -> ("Tick Count(uSec)"=w382:u32)
  }
  n206 = while "Selection" {
    stop <- FALSE stop-if-true
    # "T = Mag. encoder\nF = Motor encoder"
    n207 = case shown="1" "Vp. Est." {
      tunnel: [w418 w419 w422] -> w394
      tunnel: [w417 w420 w421] -> w395
      frame 0, Default {
        # "T"
        n208 = local read "omega_p (T)"() -> (w418:fxp<+/-,36,13>)
        n209 = local read "Dp_d (T)"() -> (w417:fxp<+/-,36,13>)
      }
      frame 1 {
        # "Mavg"
        n210 = local read "omega_p (Mavg)"() -> (w419:fxp<+/-,36,13>)
        n211 = local read "Dp_d (Mavg)"() -> (w420:fxp<+/-,36,13>)
      }
      frame 2 {
        # "Mavg w. f."
        n212 = local read "omega_p (Mavg w. f)"() -> (w422:fxp<+/-,36,14>)
        n213 = local read "Dp_d (Mavg w. f.)"() -> (w421:fxp<+/-,36,14>)
      }
    }
    "Dp_d (mm/s)" <- w395
    "omega_p (rad/s)" <- w394
    n214 = case shown="2" "Strain selection_p" {
      tunnel: [w424 w425 w426] -> w401
      frame 0, Default {
        n215 = local read "Raw Strain_p"() -> (w424:fxp<+/-,36,4>)
      }
      frame 1 {
        n216 = local read "Strain_p (Avg8)"() -> (w425:fxp<+/-,36,4>)
      }
      frame 2 {
        n217 = local read "Strain_p (Avg8 w. f)"() -> (w426:fxp<+/-,36,8>)
      }
    }
    n218 = Divide(x=w401, y="S/F coeff_p") -> (x/y=w398:fxp<+/-,32,10>)
    n219 = case shown="True" "Zero_p" {
      tunnel: w398 -> [_ w423]
      frame False {
      }
      frame True {
        "Fp_dc" <- w423
      }
    }
    n220 = local read "Fp_dc"() -> (w396:fxp<+/-,32,10>)
    n221 = Subtract(x=w398, y=w396) -> (x-y=→"Force_p":fxp<+/-,33,11>)
    n222 = case shown="True" "Mag. encoder_p" {
      tunnel: [w409 w416] -> w390
      tunnel: [w408 w415] -> w391
      tunnel: [w407 w414] -> w392
      tunnel: [w405 w413] -> w388
      tunnel: [w406 w412] -> w387
      tunnel: [w404 w410] -> w386
      tunnel: [w403 w411] -> w385
      frame False {
        n223 = local read "Encoder Position_p1"() -> (w407:i32)
        n224 = local read "rad_p1"() -> (w408:fxp<+/-,33,20>)
        n225 = local read "omega_p1 (Mavg)"() -> (w403:fxp<+/-,36,14>)
        n226 = local read "omega_p1 (T)"() -> (w405:fxp<+/-,36,13>)
        n227 = local read "D_p1"() -> (w409:fxp<+/-,32,7>)
        n228 = local read "Dp1_d (Mavg)"() -> (w404:fxp<+/-,36,14>)
        n229 = local read "Dp1_d (T)"() -> (w406:fxp<+/-,36,13>)
      }
      frame True {
        n230 = local read "Encoder Position_p2"() -> (w414:i32)
        n231 = local read "omega_p2 (Mavg)"() -> (w411:fxp<+/-,36,14>)
        n232 = local read "rad_p2"() -> (w415:fxp<+/-,33,20>)
        n233 = local read "D_p2"() -> (w416:fxp<+/-,32,7>)
        n234 = local read "Dp2_d (Mavg)"() -> (w410:fxp<+/-,36,14>)
        n235 = local read "omega_p2 (T)"() -> (w413:fxp<+/-,36,13>)
        n236 = local read "Dp2_d (T)"() -> (w412:fxp<+/-,36,13>)
      }
    }
    "D_p(mm)" <- w390
    "rad_p(NrTheta)" <- w391
    "Encoder Position_p" <- w392
    "Dp_d (T)" <- w387
    "omega_p (T)" <- w388
    "Dp_d (Mavg)" <- w386
    "omega_p (Mavg)" <- w385
  }
  n237 = while "Omega_p2 (Mavg)" {
    shift-right: [w428] -> _
    shift-left: w4 -> [w449]
    shift-right: [w429] -> _
    shift-left: w3 -> [w447]
    shift-right: [w433] -> _
    shift-left: _ -> [w431]
    tunnel: w2 -> [w445]
    tunnel: w1 -> [w450]
    stop <- FALSE stop-if-true
    w434 = fxp<+/-,27,3> 3.1415926814079285  # pi
    w437 = fxp<+,32,0> 0.1953125  # 800/4096
    w442 = fxp<+/-,32,0> 0.3183098859153688  # L/2/pi
    n238 = call "Tick Count9"() -> ("Tick Count(uSec)"=w444:u32)
    n239 = Index Array(array=w447, index=0) -> (element=w446:i32)
    n240 = Index Array(array=w449, index=0) -> (element=w448:i32)
    n241 = Multiply(x=w445, y=w450) -> (x*y=w453:i32)
    n242 = Add(x=w453, y=w446) -> (x+y=w452:i32)
    n243 = Greater Or Equal?(x=w444, y=w452) -> (x >= y?=w451:bool)
    n244 = case shown="True" w451 {
      tunnel: w449 -> [w457 w472]
      tunnel: w448 -> [_ w464]
      tunnel: w447 -> [w458 w473]
      tunnel: w446 -> [_ w474]
      tunnel: w445 -> [_ w471]
      tunnel: w444 -> [_ w459]
      tunnel: [w457 w462] -> w428
      tunnel: [w458 w461] -> w429
      tunnel: [w456 w460] -> w433
      tunnel: w431 -> [w456 _]
      frame False {
      }
      frame True {
        n245 = local read "Encoder Position_p2"() -> (w463:i32)
        n246 = Subtract(x=w459, y=w474) -> (x-y=w475:u32)
        n247 = Insert Into Array(array=w473, new element=w459) -> (w477:i32[])  [unwired: 1 in]
        n248 = Subtract(x=w463, y=w464) -> (x-y=w468:i32)
        n249 = Insert Into Array(array=w472, index=w471, new element=w463) -> (w478:i32[])
        n250 = To Fixed-Point(number=w475) -> (fixed-point=w465:fxp<+,32,32>)  [unwired: 1 in]
        n251 = Multiply(x=w468, y=2500) -> (x*y=w469:i32)
        n252 = To Fixed-Point(number=w469) -> (fixed-point=w470:fxp<+/-,32,32>)  [unwired: 1 in]
        n253 = Delete From Array(array=w477, length=1, index=0) -> (array with subset deleted=w461:i32[])  [unwired: 1 out]
        n254 = Delete From Array(array=w478, length=1, index=0) -> (array with subset deleted=w462:i32[])  [unwired: 1 out]
        n255 = Divide(x=w470, y=w465) -> (x/y=w460:fxp<+/-,64,32>)
      }
    }
    n256 = local read "Mag. factor_p"() -> (w436:fxp<+/-,20,3>)
    n257 = local read "Belt_in_p"() -> (w439:fxp<+/-,6,6>)
    n258 = local read "Belt_out_p"() -> (w438:fxp<+/-,7,7>)
    n259 = Divide(x=w437, y=w436) -> (x/y=w427:fxp<+/-,32,1>)
    n260 = Multiply(x=w434, y=w433) -> (x*y=w435:fxp<+/-,64,35>)
    n261 = Multiply(x=w442, y=w439) -> (x*y=w443:fxp<+/-,38,6>)
    n262 = Multiply(x=w427, y=w435) -> (x*y=w430:fxp<+/-,64,36>)
    "omega_p2 (Mavg)" <- w430
    n263 = Divide(x=w443, y=w438) -> (x/y=w441:fxp<+/-,45,6>)
    n264 = Multiply(x=w441, y=w430) -> (x*y=→"Dp2_d (Mavg)":fxp<+/-,64,41>)
  }
  n265 = while "Omega_p1 (Mavg)" {
    tunnel: w8 -> [w499]
    shift-right: [w497] -> _
    shift-left: w7 -> [w502]
    shift-right: [w496] -> _
    shift-left: w6 -> [w498]
    shift-right: [w495] -> _
    shift-left: _ -> [w494]
    tunnel: w5 -> [w492]
    stop <- FALSE stop-if-true
    w486 = fxp<+/-,27,3> 3.1415926814079285  # pi
    w485 = fxp<+/-,32,0> 0.3183098859153688  # L/2/pi
    n266 = call "Tick Count5"() -> ("Tick Count(uSec)"=w503:u32)
    n267 = Index Array(array=w502, index=0) -> (element=w501:u32)
    n268 = Index Array(array=w498, index=0) -> (element=w500:i32)
    n269 = Multiply(x=w499, y=w492) -> (x*y=w505:i32)
    n270 = Add(x=w505, y=w501) -> (x+y=w504:u32)
    n271 = Greater Or Equal?(x=w503, y=w504) -> (x >= y?=w493:bool)
    n272 = case shown="True" w493 {
      tunnel: w503 -> [_ w526]
      tunnel: w499 -> [_ w523]
      tunnel: w502 -> [w510 w525]
      tunnel: w501 -> [_ w524]
      tunnel: w500 -> [_ w520]
      tunnel: w498 -> [w509 w522]
      tunnel: [w508 w518] -> w495
      tunnel: [w510 w517] -> w497
      tunnel: [w509 w516] -> w496
      tunnel: w494 -> [w508 _]
      frame False {
      }
      frame True {
        n273 = local read "Encoder Position_p1"() -> (w519:i32)
        n274 = Subtract(x=w526, y=w524) -> (x-y=w527:u32)
        n275 = Subtract(x=w519, y=w520) -> (x-y=w512:i32)
        n276 = Insert Into Array(array=w525, new element=w526) -> (w529:u32[])  [unwired: 1 in]
        n277 = Insert Into Array(array=w522, index=w523, new element=w519) -> (w530:i32[])
        n278 = To Fixed-Point(number=w527) -> (fixed-point=w514:fxp<+,32,32>)  [unwired: 1 in]
        n279 = Multiply(x=w512, y=2500) -> (x*y=w513:i32)
        n280 = To Fixed-Point(number=w513) -> (fixed-point=w521:fxp<+/-,32,32>)  [unwired: 1 in]
        n281 = Delete From Array(array=w529, length=1, index=0) -> (array with subset deleted=w517:u32[])  [unwired: 1 out]
        n282 = Delete From Array(array=w530, length=1, index=0) -> (array with subset deleted=w516:i32[])  [unwired: 1 out]
        n283 = Divide(x=w521, y=w514) -> (x/y=w518:fxp<+/-,64,32>)
      }
    }
    n284 = local read "Belt_in_p"() -> (w490:fxp<+/-,6,6>)
    n285 = local read "Belt_out_p"() -> (w489:fxp<+/-,7,7>)
    n286 = Multiply(x=w486, y=w495) -> (x*y=w491:fxp<+/-,64,35>)
    n287 = Multiply(x=w485, y=w490) -> (x*y=w488:fxp<+/-,38,6>)
    n288 = Multiply(x=fxp<+/-,2,2> 1.0 ("f"), y=w491) -> (x*y=w484:fxp<+/-,64,37>)
    "omega_p1 (Mavg)" <- w484
    n289 = Divide(x=w488, y=w489) -> (x/y=w483:fxp<+/-,45,6>)
    n290 = Multiply(x=w483, y=w484) -> (x*y=→"Dp1_d (Mavg)":fxp<+/-,64,42>)
  }
  n291 = while "Quadrature drive_p" {
    stop <- FALSE stop-if-true
    n292 = local read "Drive mode"() -> (w534:i16)
    n293 = case shown="1" w534 {
      tunnel: [w544 w545] -> w533
      frame 0, Default {
        # "Backward"
        n294 = local read "Fp_PID"() -> (w544:fxp<+/-,36,16>)
      }
      frame 1 {
        # "Forward"
        n295 = local read "Fr_p"() -> (w545:fxp<+/-,32,10>)
      }
    }
    n296 = local read "dFp_PID"() -> (w537:fxp<+/-,36,18>)
    n297 = local read "omega_p (rad/s)"() -> (w541:fxp<+/-,36,13>)
    n298 = Select(t=w537, s="dFp_add", f=fxp<+,1,1> 0.0) -> (s? t:f=w540:fxp<+/-,36,18>)
    n299 = call "Oriental_step_motor_PKP225.vi"("F_Threshold"="F_Threshold_p", "dFmr"=w540, "omega"=w541, "Fmr"=w533) -> ("vq_F"=→"vq_p_F":fxp<+/-,36,9>, "vd_F"=→"vd_p_F":fxp<+/-,36,9>)  [unwired: 6 in]
  }
  n300 = while "PID force controller_p" {
    shift-right: [w550] -> _
    shift-left: _ -> [w549]
    stop <- FALSE stop-if-true
    n301 = local read "Force_p"() -> (w562:fxp<+/-,32,10>)
    n302 = local read "fpt_d"() -> (w558:fxp<+/-,36,18>)
    n303 = local read "Fr_p"() -> (w563:fxp<+/-,32,10>)
    n304 = Subtract(x=w563, y=w562) -> (x-y=w560:fxp<+/-,33,11>)
    "fp_tilde" <- w560
    n305 = local read "fpt_i"() -> (w554:fxp<+/-,34,18>)
    n306 = Multiply(x="Kp_p", y=w560) -> (x*y=w556:fxp<+/-,64,23>)
    n307 = Multiply(x="Kd_p", y=w558) -> (x*y=w557:fxp<+/-,64,27>)
    n308 = Absolute Value(x=w560) -> (abs(x)=w569:fxp<+,32,10>)
    n309 = Add(x=w556, y=w557) -> (x+y=w552:fxp<+/-,64,28>)
    n310 = Multiply(x="Ki_p", y=w554) -> (x*y=w553:fxp<+/-,64,27>)
    n311 = call "Tick Count7"() -> ("Tick Count(uSec)"=w550:u32)
    n312 = Add(x=w552, y=w553) -> (x+y=w551:fxp<+/-,64,29>)
    n313 = Greater?(x=w569, y="fp_tolorance") -> (0:w566:bool)
    n314 = Subtract(x=w550, y=w549) -> (x-y=w548:u32)
    n315 = Divide(x=u32 1000, y=w548) -> (x/y=→"PID (kHz)":fxp<+/-,20,7>)
    n316 = Select(t=w551, s=w566, f=fxp<+,1,1> 0.0) -> (s? t:f=→"Fp_PID":fxp<+/-,64,29>)
  }
  n317 = while "ft_d" {
    stop <- FALSE stop-if-true
    n318 = local read "Dp_error_dd"() -> (w576:fxp<+/-,36,16>)
    n319 = local read "Dp_error_d"() -> (w578:fxp<+/-,33,8>)
    n320 = local read "Kv_p"() -> (w579:fxp<+/-,22,8>)
    n321 = local read "Bv_p"() -> (w577:fxp<+/-,22,8>)
    n322 = Multiply(x=w578, y=w579) -> (x*y=w574:fxp<+/-,55,16>)
    n323 = Multiply(x=w576, y=w577) -> (x*y=w575:fxp<+/-,58,24>)
    n324 = local read "Force_p"() -> (w572:fxp<+/-,32,10>)
    n325 = Add(x=w574, y=w575) -> (x+y=w573:fxp<+/-,63,24>)
    n326 = Subtract(x=w573, y=w572) -> (x-y=→"fpt_d":fxp<+/-,63,24>)
  }
  n327 = while "Derivative" {
    stop <- FALSE stop-if-true
    n328 = local read "Dpr_sin_dd"() -> (w588:fxp<+/-,35,20>)
    n329 = local read "Dpr_sin_d"() -> (w590:fxp<+/-,33,15>)
    n330 = local read "Stop motor_p"() -> (w586:bool)
    n331 = local read "Dp_error"() -> (w591:fxp<+/-,22,7>)
    n332 = local read "Dp_dd"() -> (w589:fxp<+/-,36,25>)
    n333 = Subtract(x=w590, y=w591) -> (x-y=w583:fxp<+/-,34,16>)
    n334 = Subtract(x=w588, y=w589) -> (x-y=w587:fxp<+/-,41,26>)
    n335 = Select(t=fxp<+,1,1> 0.0, s=w586, f=w583) -> (s? t:f=→"Dp_error_d":fxp<+/-,34,16>)
    n336 = Select(t=fxp<+/-,41,26> 0.0, s=w586, f=w587) -> (s? t:f=→"Dp_error_dd":fxp<+/-,41,26>)
  }
  n337 = xnode "FPGA I/O Node"("error in"=w9, "Mod6/Stop"=TRUE) -> ()  [unwired: 1 in, 2 out]
  n338 = while {
    stop <- FALSE stop-if-true
    n339 = local read "omega_p1 (Mavg)"() -> (w598:fxp<+/-,36,14>)
    n340 = local read "Dp1_d (Mavg)"() -> (w594:fxp<+/-,36,14>)
    n341 = xnode "Butterworth Filter"("input data"=w598, "scaled coefficients"="omega_P(Mavg) coeff.") -> ("output data"=→"omega_p (Mavg w. f)":fxp<+/-,36,18>)  [unwired: 1 in]
    n342 = xnode "Butterworth Filter"("input data"=w594, "scaled coefficients"="Dp_d (Mavg) coeff.") -> ("output data"=→"Dp_d (Mavg w. f.)":fxp<+/-,36,18>)  [unwired: 1 in]
  }
